vi "Lab Panel V6.00.vi"() -> ()   [LabVIEW 2017] (continued)
                  tunnel: [w1483 w1515] -> w1477
                  tunnel: w1475 -> [_ w1514]
                  tunnel: w1474 -> [_ w1513]
                  tunnel: w1473 -> [_ w1512]
                  tunnel: w1472 -> [_ w1510]
                  frame False {
                    # "stop test"
                    n865 = stacked-sequence {
                      tunnel: w1484 -> [w1493 _]
                      tunnel: [w1485 _] -> w1483
                      frame #0 {
                        n866 = local read "DISP LAB03-2"() -> (w1492:T4)
                        n867 = Unbundle(w1492) -> ("CYCLE"=w1490:dbl, "MINS"=w1491:dbl)  [unwired: 1 out]
                        n868 = case shown="\"CYCLE TEST\"" w1493 {
                          tunnel: w1491 -> [_ _ w1500]
                          tunnel: w1490 -> [w1498 w1499 _]
                          tunnel: [w1498 w1499 w1500] -> w1489
                          frame "CHART TEST", Default {
                          }
                          frame "CYCLE TEST" {
                          }
                          frame "T-RISE TEST" {
                          }
                        }
                        n869 = local read "TDMS LAB03-2"() -> (w1497:refnum<k34>)
                        n870 = Build Array("STOPPED") -> (w1494:string[])
                        n871 = Build Array(w1489) -> (w1488:dbl[])
                        n872 = TDMS Write(0:w1497, 5:"TEST RESULT", 7:w1494, 9:w1488) -> (4:w1486:refnum<k34>, 15:w1487:errorcluster)  [unwired: 2 in, 2 out]
                        n873 = TDMS Close(8:w1487, 11:w1486) -> (0:w1485:errorcluster)  [unwired: 1 out]
                      }
                      frame #1 {
                        n874 = local read "DISP LAB03-2"() -> (w1504:T4)
                        n875 = stacked-sequence {
                          tunnel: "LAB03-2" -> [w1506 w1508]
                          frame #0 {
                            n876 = call "sub vi - defrag tdms v1.vi"("panel id"=w1506) -> ("error out"=w1505:errorcluster)  [unwired: 10 in]
                            n877 = local write "data file error"(w1505) -> ()
                          }
                          frame #1 {
                            n878 = call "Save data file (stop) v3.vi"("panel id"=w1508) -> ("network file save error"=w1507:errorcluster)  [unwired: 9 in, 1 out]
                            n879 = local write "RESULT LAB03-2"(FALSE) -> ()
                            n880 = local write "data file error"(w1507) -> ()
                          }
                        }
                        n881 = Bundle(cluster=w1504, "STATUS"="STOP") -> (w1502:T4)  [unwired: 2 in]
                        n882 = local write "DISP LAB03-2"(w1502) -> ()
                      }
                    }
                  }
                  frame True {
                    n883 = local read "SIG LAB03-2"() -> (w1511:T2)
                    n884 = stacked-sequence {
                      seq-local: [w1522 _] -> [_ w1526]
                      tunnel: w1520 -> [_ w1536]
                      tunnel: w1519 -> [_ w1535]
                      tunnel: w1518 -> [_ w1534]
                      tunnel: w1517 -> [_ w1533]
                      tunnel: w1516 -> [_ w1532]
                      tunnel: [_ w1531] -> w1515
                      tunnel: w1514 -> [_ w1530]
                      tunnel: w1513 -> [_ w1529]
                      tunnel: w1512 -> [_ w1528]
                      tunnel: w1511 -> [w1521 w1527]
                      tunnel: w1510 -> [_ w1525]
                      frame #0 {
                        n885 = Unbundle(w1521) -> ("AMPS"=w1524:dbl)  [unwired: 4 out]
                        n886 = call "Check For Amps on v1.vi"("ID"="LAB03-2", "amps"=w1524) -> ("amps"=w1522:bool)  [unwired: 9 in]
                      }
                      frame #1 {
                        n887 = case shown="True" w1526 {
                          tunnel: w1536 -> [_ w1549]
                          tunnel: w1535 -> [_ w1548]
                          tunnel: w1534 -> [_ w1547]
                          tunnel: w1533 -> [_ w1546]
                          tunnel: w1532 -> [_ w1545]
                          tunnel: [errorcluster {"status"=FALSE, "code"=0, "source"=""} ("error out") w1544] -> w1531
                          tunnel: w1530 -> [_ w1543]
                          tunnel: w1529 -> [_ w1542]
                          tunnel: w1528 -> [_ w1541]
                          tunnel: w1527 -> [_ w1540]
                          tunnel: w1525 -> [_ w1539]
                          frame False {
                            w1537 = FALSE
                            n888 = local write "RUN LAB03-2"(w1537) -> ()
                            n889 = local write "run lab03-2"(w1537) -> ()
                          }
                          frame True {
                            n890 = stacked-sequence {
                              seq-local: [w1550 _ _ _ _] -> [_ w1574 _ _ _]
                              tunnel: w1549 -> [w1555 _ _ _ _]
                              tunnel: w1548 -> [w1552 _ _ _ _]
                              tunnel: w1547 -> [w1565 _ _ _ _]
                              tunnel: w1546 -> [w1558 _ _ _ _]
                              tunnel: w1545 -> [w1553 _ _ _ _]
                              tunnel: [_ w1569 _ _ _] -> w1544
                              tunnel: w1543 -> [_ _ _ w1595 _]
                              tunnel: w1542 -> [_ _ _ w1594 _]
                              tunnel: w1541 -> [_ _ _ w1593 _]
                              tunnel: w1540 -> [_ _ _ _ _]
                              tunnel: w1539 -> [_ _ _ _ w1609]
                              frame #0 {
                                w1551 = "\\"
                                n891 = local read "SET LAB03-2"() -> (w1560:T5)
                                n892 = case shown="\"T-RISE TEST\"" w1565 {
                                tunnel: ["L03-2-CHART TEST-" "L03-2-CYCLE TEST-" "L03-2-T-RISE TEST-"] -> w1561
                                frame "CHART TEST", Default {
                                }
                                frame "CYCLE TEST" {
                                }
                                frame "T-RISE TEST" {
                                }
                                }
                                n893 = Unbundle(w1560) -> ("DESCRIPTION"=w1559:string)  [unwired: 4 out]
                                n894 = Concatenate Strings(w1555, "\\", w1553, w1551, w1552, w1551) -> (w1562:string)
                                n895 = String To Path(string=w1562) -> (path=w1564:path)
                                n896 = Concatenate Strings(w1562, w1561, w1559, "-", w1558, ".tdms") -> (w1550:string)
                                n897 = Create Folder(path (use dialog)=w1564) -> (error out=w1563:errorcluster)  [unwired: 2 in, 2 out]
                                n898 = global write "Global 1.vi" "LAB03-2 FILE"(w1550) -> ()
                                n899 = call <vilib>:"Clear Errors.vi"("error in (no error)"=w1563) -> ()  [unwired: 5 in, 2 out]
                              }
                              frame #1 {
                                (unwired) FALSE
                                n900 = String To Path(string=w1574) -> (path=w1570:path)
                                n901 = TDMS Open(6:FALSE, 10:T22."create or replace" ("operation (0:open)"), 11:w1570) -> (0:w1569:errorcluster, 3:→"TDMS LAB03-2":refnum<k34>)  [unwired: 4 in]
                              }
                              frame #2 {
                                n902 = local read "SET LAB03-2"() -> (w1580:T5)
                                n903 = local read "TDMS LAB03-2"() -> (w1591:refnum<k34>)
                                n904 = Build Array("Testers Name", "Description", "Set Test Cycles", "T-Rise minutes", "T-Rise Deg C") -> (w1581:string[])
                                n905 = Unbundle(w1580) -> ("NAME"=w1579:string, "DESCRIPTION"=w1578:string, "CYCLES"=w1577:dbl, "T-RISE mins"=w1576:dbl, "T-RISE deg C"=w1575:dbl)
                                n906 = Number To Decimal String(number=w1577) -> (decimal integer string=w1590:string)  [unwired: 1 in]
                                n907 = Number To Decimal String(number=w1576) -> (decimal integer string=w1589:string)  [unwired: 1 in]
                                n908 = Number To Decimal String(number=w1575) -> (decimal integer string=w1588:string)  [unwired: 1 in]
                                n909 = Build Array(w1579, w1578, w1590, w1589, w1588) -> (w1587:string[])
                                n910 = TDMS Set Properties(5:w1587, 7:w1581, 11:w1591) -> ()  [unwired: 3 in, 4 out]
                              }
                              frame #3 {
                                n911 = local read "DISP LAB03-2"() -> (w1596:T4)
                                n912 = Concatenate Strings("LAB03-2  ", w1595) -> (w1597:string)
                                n913 = Two Button Dialog(message=w1597, 1:w1593, 2:w1594) -> (T button?=w1599:bool)
                                n914 = case shown="True" w1599 {
                                tunnel: w1596 -> [w1606 w1607]
                                tunnel: [w1606 w1607] -> w1603
                                tunnel: [w1605 w1608] -> w1602
                                tunnel: [w1604 w1608] -> w1601
                                frame False {
                                n915 = Unbundle(w1606) -> ("CYCLE"=w1605:dbl, "MINS"=w1604:dbl)  [unwired: 1 out]
                                }
                                frame True {
                                w1608 = 0.0
                                }
                                }
                                n916 = Bundle(cluster=w1603, "CYCLE"=w1602, "MINS"=w1601, "STATUS"="RUN") -> (w1592:T4)
                                n917 = local write "DISP LAB03-2"(w1592) -> ()
                              }
                              frame #4 {
                                n918 = local read "TEMP START LAB03-2"() -> (w1611:cluster{"TL":dbl, "TN":dbl})
                                n919 = Bundle(cluster=w1611, "TL"=w1609, "TN"=w1609) -> (w1610:cluster{"TL":dbl, "TN":dbl})
                                n920 = local write "TEMP START LAB03-2"(w1610) -> ()
                              }
                            }
                          }
                        }
                      }
                    }
                  }
                }
              }
              event "RUN LAB04-1": Value Change {
                n921 = event-data() -> ("NewVal"=w1616:bool)  [unwired: 1 in, 5 out]
                n922 = local write "run lab04-1"(w1616) -> ()
                n923 = case shown="True" w1616 {
                  tunnel: w1622 -> [_ w1660]
                  tunnel: w1621 -> [_ w1659]
                  tunnel: w1619 -> [w1624 w1658]
                  tunnel: w1620 -> [_ w1657]
                  tunnel: w1618 -> [_ w1656]
                  tunnel: [w1623 w1655] -> w1617
                  tunnel: w1615 -> [_ w1654]
                  tunnel: w1614 -> [_ w1653]
                  tunnel: w1613 -> [_ w1652]
                  tunnel: w1612 -> [_ w1650]
                  frame False {
                    # "stop test"
                    n924 = stacked-sequence {
                      tunnel: w1624 -> [w1633 _]
                      tunnel: [w1625 _] -> w1623
                      frame #0 {
                        n925 = local read "DISP LAB04-1"() -> (w1632:T4)
                        n926 = Unbundle(w1632) -> ("CYCLE"=w1630:dbl, "MINS"=w1631:dbl)  [unwired: 1 out]
                        n927 = case shown="\"CYCLE TEST\"" w1633 {
                          tunnel: w1631 -> [_ _ w1640]
                          tunnel: w1630 -> [w1638 w1639 _]
                          tunnel: [w1638 w1639 w1640] -> w1629
                          frame "CHART TEST", Default {
                          }
                          frame "CYCLE TEST" {
                          }
                          frame "T-RISE TEST" {
                          }
                        }
                        n928 = local read "TDMS LAB04-1"() -> (w1637:refnum<k34>)
                        n929 = Build Array("STOPPED") -> (w1634:string[])
                        n930 = Build Array(w1629) -> (w1628:dbl[])
                        n931 = TDMS Write(0:w1637, 5:"TEST RESULT", 7:w1634, 9:w1628) -> (4:w1626:refnum<k34>, 15:w1627:errorcluster)  [unwired: 2 in, 2 out]
                        n932 = TDMS Close(8:w1627, 11:w1626) -> (0:w1625:errorcluster)  [unwired: 1 out]
                      }
                      frame #1 {
                        n933 = local read "DISP LAB04-1"() -> (w1644:T4)
                        n934 = stacked-sequence {
                          tunnel: "LAB04-1" -> [w1646 w1648]
                          frame #0 {
                            n935 = call "sub vi - defrag tdms v1.vi"("panel id"=w1646) -> ("error out"=w1645:errorcluster)  [unwired: 10 in]
                            n936 = local write "data file error"(w1645) -> ()
                          }
                          frame #1 {
                            n937 = call "Save data file (stop) v3.vi"("panel id"=w1648) -> ("network file save error"=w1647:errorcluster)  [unwired: 9 in, 1 out]
                            n938 = local write "RESULT LAB04-1"(FALSE) -> ()
                            n939 = local write "data file error"(w1647) -> ()
                          }
                        }
                        n940 = Bundle(cluster=w1644, "STATUS"="STOP") -> (w1642:T4)  [unwired: 2 in]
                        n941 = local write "DISP LAB04-1"(w1642) -> ()
                      }
                    }
                  }
                  frame True {
                    n942 = local read "SIG LAB04-1"() -> (w1651:T2)
                    n943 = stacked-sequence {
                      seq-local: [w1662 _] -> [_ w1666]
                      tunnel: w1660 -> [_ w1676]
                      tunnel: w1659 -> [_ w1675]
                      tunnel: w1658 -> [_ w1674]
                      tunnel: w1657 -> [_ w1673]
                      tunnel: w1656 -> [_ w1672]
                      tunnel: [_ w1671] -> w1655
                      tunnel: w1654 -> [_ w1670]
                      tunnel: w1653 -> [_ w1669]
                      tunnel: w1652 -> [_ w1668]
                      tunnel: w1651 -> [w1661 w1667]
                      tunnel: w1650 -> [_ w1665]
                      frame #0 {
                        n944 = Unbundle(w1661) -> ("AMPS"=w1664:dbl)  [unwired: 4 out]
                        n945 = call "Check For Amps on v1.vi"("ID"="LAB04-1", "amps"=w1664) -> ("amps"=w1662:bool)  [unwired: 9 in]
                      }
                      frame #1 {
                        n946 = case shown="True" w1666 {
                          tunnel: w1676 -> [_ w1689]
                          tunnel: w1675 -> [_ w1688]
                          tunnel: w1674 -> [_ w1687]
                          tunnel: w1673 -> [_ w1686]
                          tunnel: w1672 -> [_ w1685]
                          tunnel: [errorcluster {"status"=FALSE, "code"=0, "source"=""} ("error out") w1684] -> w1671
                          tunnel: w1670 -> [_ w1683]
                          tunnel: w1669 -> [_ w1682]
                          tunnel: w1668 -> [_ w1681]
                          tunnel: w1667 -> [_ w1680]
                          tunnel: w1665 -> [_ w1679]
                          frame False {
                            w1677 = FALSE
                            n947 = local write "RUN LAB04-1"(w1677) -> ()
                            n948 = local write "run lab04-1"(w1677) -> ()
                          }
                          frame True {
                            n949 = stacked-sequence {
                              seq-local: [w1690 _ _ _ _] -> [_ w1714 _ _ _]
                              tunnel: w1689 -> [w1695 _ _ _ _]
                              tunnel: w1688 -> [w1691 _ _ _ _]
                              tunnel: w1687 -> [w1705 _ _ _ _]
                              tunnel: w1686 -> [w1698 _ _ _ _]
                              tunnel: w1685 -> [w1693 _ _ _ _]
                              tunnel: [_ w1709 _ _ _] -> w1684
                              tunnel: w1683 -> [_ _ _ w1735 _]
                              tunnel: w1682 -> [_ _ _ w1734 _]
                              tunnel: w1681 -> [_ _ _ w1733 _]
                              tunnel: w1680 -> [_ _ _ _ _]
                              tunnel: w1679 -> [_ _ _ _ w1749]
                              frame #0 {
                                w1692 = "\\"
                                n950 = local read "SET LAB04-1"() -> (w1700:T5)
                                n951 = case shown="\"CYCLE TEST\"" w1705 {
                                tunnel: ["L04-1-CHART TEST-" "L04-1-CYCLE TEST-" "L04-1-T-RISE TEST-"] -> w1701
                                frame "CHART TEST", Default {
                                }
                                frame "CYCLE TEST" {
                                }
                                frame "T-RISE TEST" {
                                }
                                }
                                n952 = Unbundle(w1700) -> ("DESCRIPTION"=w1699:string)  [unwired: 4 out]
                                n953 = Concatenate Strings(w1695, "\\", w1693, w1692, w1691, w1692) -> (w1702:string)
                                n954 = String To Path(string=w1702) -> (path=w1704:path)
                                n955 = Concatenate Strings(w1702, w1701, w1699, "-", w1698, ".tdms") -> (w1690:string)
                                n956 = Create Folder(path (use dialog)=w1704) -> (error out=w1703:errorcluster)  [unwired: 2 in, 2 out]
                                n957 = global write "Global 1.vi" "LAB04-1 FILE"(w1690) -> ()
                                n958 = call <vilib>:"Clear Errors.vi"("error in (no error)"=w1703) -> ()  [unwired: 5 in, 2 out]
                              }
                              frame #1 {
                                (unwired) FALSE
                                n959 = String To Path(string=w1714) -> (path=w1710:path)
                                n960 = TDMS Open(6:FALSE, 10:T22."create or replace" ("operation (0:open)"), 11:w1710) -> (0:w1709:errorcluster, 3:→"TDMS LAB04-1":refnum<k34>)  [unwired: 4 in]
                              }
                              frame #2 {
                                n961 = local read "SET LAB04-1"() -> (w1720:T5)
                                n962 = local read "TDMS LAB04-1"() -> (w1731:refnum<k34>)
                                n963 = Build Array("Testers Name", "Description", "Set Test Cycles", "T-Rise minutes", "T-Rise Deg C") -> (w1721:string[])
                                n964 = Unbundle(w1720) -> ("NAME"=w1719:string, "DESCRIPTION"=w1718:string, "CYCLES"=w1717:dbl, "T-RISE mins"=w1716:dbl, "T-RISE deg C"=w1715:dbl)
                                n965 = Number To Decimal String(number=w1717) -> (decimal integer string=w1730:string)  [unwired: 1 in]
                                n966 = Number To Decimal String(number=w1716) -> (decimal integer string=w1729:string)  [unwired: 1 in]
                                n967 = Number To Decimal String(number=w1715) -> (decimal integer string=w1728:string)  [unwired: 1 in]
                                n968 = Build Array(w1719, w1718, w1730, w1729, w1728) -> (w1727:string[])
                                n969 = TDMS Set Properties(5:w1727, 7:w1721, 11:w1731) -> ()  [unwired: 3 in, 4 out]
                              }
                              frame #3 {
                                n970 = local read "DISP LAB04-1"() -> (w1736:T4)
                                n971 = Concatenate Strings("LAB04-1  ", w1735) -> (w1737:string)
                                n972 = Two Button Dialog(message=w1737, 1:w1733, 2:w1734) -> (T button?=w1739:bool)
                                n973 = case shown="True" w1739 {
                                tunnel: w1736 -> [w1746 w1747]
                                tunnel: [w1746 w1747] -> w1743
                                tunnel: [w1745 w1748] -> w1742
                                tunnel: [w1744 w1748] -> w1741
                                frame False {
                                n974 = Unbundle(w1746) -> ("CYCLE"=w1745:dbl, "MINS"=w1744:dbl)  [unwired: 1 out]
                                }
                                frame True {
                                w1748 = 0.0
                                }
                                }
                                n975 = Bundle(cluster=w1743, "CYCLE"=w1742, "MINS"=w1741, "STATUS"="RUN") -> (w1732:T4)
                                n976 = local write "DISP LAB04-1"(w1732) -> ()
                              }
                              frame #4 {
                                n977 = local read "TEMP START LAB04-1"() -> (w1751:cluster{"TL":dbl, "TN":dbl})
                                n978 = Bundle(cluster=w1751, "TL"=w1749, "TN"=w1749) -> (w1750:cluster{"TL":dbl, "TN":dbl})
                                n979 = local write "TEMP START LAB04-1"(w1750) -> ()
                              }
                            }
                          }
                        }
                      }
                    }
                  }
                }
              }
              event "RUN LAB04-2": Value Change {
                n980 = event-data() -> ("NewVal"=w1756:bool)  [unwired: 1 in, 5 out]
                n981 = local write "run lab04-2"(w1756) -> ()
                n982 = case shown="True" w1756 {
                  tunnel: w1762 -> [_ w1800]
                  tunnel: w1761 -> [_ w1799]
                  tunnel: w1759 -> [w1764 w1798]
                  tunnel: w1760 -> [_ w1797]
                  tunnel: w1758 -> [_ w1796]
                  tunnel: [w1763 w1795] -> w1757
                  tunnel: w1755 -> [_ w1794]
                  tunnel: w1754 -> [_ w1793]
                  tunnel: w1753 -> [_ w1792]
                  tunnel: w1752 -> [_ w1790]
                  frame False {
                    # "stop test"
                    n983 = stacked-sequence {
                      tunnel: w1764 -> [w1773 _]
                      tunnel: [w1765 _] -> w1763
                      frame #0 {
                        n984 = local read "DISP LAB04-2"() -> (w1772:T4)
                        n985 = Unbundle(w1772) -> ("CYCLE"=w1770:dbl, "MINS"=w1771:dbl)  [unwired: 1 out]
                        n986 = case shown="\"CYCLE TEST\"" w1773 {
                          tunnel: w1771 -> [_ _ w1780]
                          tunnel: w1770 -> [w1778 w1779 _]
                          tunnel: [w1778 w1779 w1780] -> w1769
                          frame "CHART TEST", Default {
                          }
                          frame "CYCLE TEST" {
                          }
                          frame "T-RISE TEST" {
                          }
                        }
                        n987 = local read "TDMS LAB04-2"() -> (w1777:refnum<k34>)
                        n988 = Build Array("STOPPED") -> (w1774:string[])
                        n989 = Build Array(w1769) -> (w1768:dbl[])
                        n990 = TDMS Write(0:w1777, 5:"TEST RESULT", 7:w1774, 9:w1768) -> (4:w1766:refnum<k34>, 15:w1767:errorcluster)  [unwired: 2 in, 2 out]
                        n991 = TDMS Close(8:w1767, 11:w1766) -> (0:w1765:errorcluster)  [unwired: 1 out]
                      }
                      frame #1 {
                        n992 = local read "DISP LAB04-2"() -> (w1784:T4)
                        n993 = stacked-sequence {
                          tunnel: "LAB04-2" -> [w1786 w1788]
                          frame #0 {
                            n994 = call "sub vi - defrag tdms v1.vi"("panel id"=w1786) -> ("error out"=w1785:errorcluster)  [unwired: 10 in]
                            n995 = local write "data file error"(w1785) -> ()
                          }
                          frame #1 {
                            n996 = call "Save data file (stop) v3.vi"("panel id"=w1788) -> ("network file save error"=w1787:errorcluster)  [unwired: 9 in, 1 out]
                            n997 = local write "RESULT LAB04-2"(FALSE) -> ()
                            n998 = local write "data file error"(w1787) -> ()
                          }
                        }
                        n999 = Bundle(cluster=w1784, "STATUS"="STOP") -> (w1782:T4)  [unwired: 2 in]
                        n1000 = local write "DISP LAB04-2"(w1782) -> ()
                      }
                    }
                  }
                  frame True {
                    n1001 = local read "SIG LAB04-2"() -> (w1791:T2)
                    n1002 = stacked-sequence {
                      seq-local: [w1802 _] -> [_ w1806]
                      tunnel: w1800 -> [_ w1816]
                      tunnel: w1799 -> [_ w1815]
                      tunnel: w1798 -> [_ w1814]
                      tunnel: w1797 -> [_ w1813]
                      tunnel: w1796 -> [_ w1812]
                      tunnel: [_ w1811] -> w1795
                      tunnel: w1794 -> [_ w1810]
                      tunnel: w1793 -> [_ w1809]
                      tunnel: w1792 -> [_ w1808]
                      tunnel: w1791 -> [w1801 w1807]
                      tunnel: w1790 -> [_ w1805]
                      frame #0 {
                        n1003 = Unbundle(w1801) -> ("AMPS"=w1804:dbl)  [unwired: 4 out]
                        n1004 = call "Check For Amps on v1.vi"("ID"="LAB04-2", "amps"=w1804) -> ("amps"=w1802:bool)  [unwired: 9 in]
                      }
                      frame #1 {
                        n1005 = case shown="True" w1806 {
                          tunnel: w1816 -> [_ w1829]
                          tunnel: w1815 -> [_ w1828]
                          tunnel: w1814 -> [_ w1827]
                          tunnel: w1813 -> [_ w1826]
                          tunnel: w1812 -> [_ w1825]
                          tunnel: [errorcluster {"status"=FALSE, "code"=0, "source"=""} ("error out") w1824] -> w1811
                          tunnel: w1810 -> [_ w1823]
                          tunnel: w1809 -> [_ w1822]
                          tunnel: w1808 -> [_ w1821]
                          tunnel: w1807 -> [_ w1820]
                          tunnel: w1805 -> [_ w1819]
                          frame False {
                            w1817 = FALSE
                            n1006 = local write "RUN LAB04-2"(w1817) -> ()
                            n1007 = local write "run lab04-2"(w1817) -> ()
                          }
                          frame True {
                            n1008 = stacked-sequence {
                              seq-local: [w1830 _ _ _ _] -> [_ w1854 _ _ _]
                              tunnel: w1829 -> [w1835 _ _ _ _]
                              tunnel: w1828 -> [w1831 _ _ _ _]
                              tunnel: w1827 -> [w1845 _ _ _ _]
                              tunnel: w1826 -> [w1838 _ _ _ _]
                              tunnel: w1825 -> [w1833 _ _ _ _]
                              tunnel: [_ w1849 _ _ _] -> w1824
                              tunnel: w1823 -> [_ _ _ w1875 _]
                              tunnel: w1822 -> [_ _ _ w1874 _]
                              tunnel: w1821 -> [_ _ _ w1873 _]
                              tunnel: w1820 -> [_ _ _ _ _]
                              tunnel: w1819 -> [_ _ _ _ w1889]
                              frame #0 {
                                w1832 = "\\"
                                n1009 = local read "SET LAB04-2"() -> (w1840:T5)
                                n1010 = case shown="\"CHART TEST\", Default" w1845 {
                                tunnel: ["L04-2-CHART TEST-" "L04-2-CYCLE TEST-" "L04-2-T-RISE TEST-"] -> w1841
                                frame "CHART TEST", Default {
                                }
                                frame "CYCLE TEST" {
                                }
                                frame "T-RISE TEST" {
                                }
                                }
                                n1011 = Unbundle(w1840) -> ("DESCRIPTION"=w1839:string)  [unwired: 4 out]
                                n1012 = Concatenate Strings(w1835, "\\", w1833, w1832, w1831, w1832) -> (w1842:string)
                                n1013 = String To Path(string=w1842) -> (path=w1844:path)
                                n1014 = Concatenate Strings(w1842, w1841, w1839, "-", w1838, ".tdms") -> (w1830:string)
                                n1015 = Create Folder(path (use dialog)=w1844) -> (error out=w1843:errorcluster)  [unwired: 2 in, 2 out]
                                n1016 = global write "Global 1.vi" "LAB04-2 FILE"(w1830) -> ()
                                n1017 = call <vilib>:"Clear Errors.vi"("error in (no error)"=w1843) -> ()  [unwired: 5 in, 2 out]
                              }
                              frame #1 {
                                (unwired) FALSE
                                n1018 = String To Path(string=w1854) -> (path=w1850:path)
                                n1019 = TDMS Open(6:FALSE, 10:T22."create or replace" ("operation (0:open)"), 11:w1850) -> (0:w1849:errorcluster, 3:→"TDMS LAB04-2":refnum<k34>)  [unwired: 4 in]
                              }
                              frame #2 {
                                n1020 = local read "SET LAB04-2"() -> (w1860:T5)
                                n1021 = local read "TDMS LAB04-2"() -> (w1871:refnum<k34>)
                                n1022 = Build Array("Testers Name", "Description", "Set Test Cycles", "T-Rise minutes", "T-Rise Deg C") -> (w1861:string[])
                                n1023 = Unbundle(w1860) -> ("NAME"=w1859:string, "DESCRIPTION"=w1858:string, "CYCLES"=w1857:dbl, "T-RISE mins"=w1856:dbl, "T-RISE deg C"=w1855:dbl)
                                n1024 = Number To Decimal String(number=w1857) -> (decimal integer string=w1870:string)  [unwired: 1 in]
                                n1025 = Number To Decimal String(number=w1856) -> (decimal integer string=w1869:string)  [unwired: 1 in]
                                n1026 = Number To Decimal String(number=w1855) -> (decimal integer string=w1868:string)  [unwired: 1 in]
                                n1027 = Build Array(w1859, w1858, w1870, w1869, w1868) -> (w1867:string[])
                                n1028 = TDMS Set Properties(5:w1867, 7:w1861, 11:w1871) -> ()  [unwired: 3 in, 4 out]
                              }
                              frame #3 {
                                n1029 = local read "DISP LAB04-2"() -> (w1876:T4)
                                n1030 = Concatenate Strings("LAB04-2 ", w1875) -> (w1877:string)
                                n1031 = Two Button Dialog(message=w1877, 1:w1873, 2:w1874) -> (T button?=w1879:bool)
                                n1032 = case shown="True" w1879 {
                                tunnel: w1876 -> [w1886 w1887]
                                tunnel: [w1886 w1887] -> w1883
                                tunnel: [w1885 w1888] -> w1882
                                tunnel: [w1884 w1888] -> w1881
                                frame False {
                                n1033 = Unbundle(w1886) -> ("CYCLE"=w1885:dbl, "MINS"=w1884:dbl)  [unwired: 1 out]
                                }
                                frame True {
                                w1888 = 0.0
                                }
                                }
                                n1034 = Bundle(cluster=w1883, "CYCLE"=w1882, "MINS"=w1881, "STATUS"="RUN") -> (w1872:T4)
                                n1035 = local write "DISP LAB04-2"(w1872) -> ()
                              }
                              frame #4 {
                                n1036 = local read "TEMP START LAB04-2"() -> (w1891:cluster{"TL":dbl, "TN":dbl})
                                n1037 = Bundle(cluster=w1891, "TL"=w1889, "TN"=w1889) -> (w1890:cluster{"TL":dbl, "TN":dbl})
                                n1038 = local write "TEMP START LAB04-2"(w1890) -> ()
                              }
                            }
                          }
                        }
                      }
                    }
                  }
                }
              }
              event "RUN LAB05-1": Value Change {
                n1039 = event-data() -> ("NewVal"=w1896:bool)  [unwired: 1 in, 5 out]
                n1040 = local write "run lab05-1"(w1896) -> ()
                n1041 = case shown="True" w1896 {
                  tunnel: w1902 -> [_ w1940]
                  tunnel: w1901 -> [_ w1939]
                  tunnel: w1899 -> [w1904 w1938]
                  tunnel: w1900 -> [_ w1937]
                  tunnel: w1898 -> [_ w1936]
                  tunnel: [w1903 w1935] -> w1897
                  tunnel: w1895 -> [_ w1934]
                  tunnel: w1894 -> [_ w1933]
                  tunnel: w1893 -> [_ w1932]
                  tunnel: w1892 -> [_ w1930]
                  frame False {
                    # "stop test"
                    n1042 = stacked-sequence {
                      tunnel: w1904 -> [w1913 _]
                      tunnel: [w1905 _] -> w1903
                      frame #0 {
                        n1043 = local read "DISP LAB05-1"() -> (w1912:T4)
                        n1044 = Unbundle(w1912) -> ("CYCLE"=w1910:dbl, "MINS"=w1911:dbl)  [unwired: 1 out]
                        n1045 = case shown="\"CYCLE TEST\"" w1913 {
                          tunnel: w1911 -> [_ _ w1920]
                          tunnel: w1910 -> [w1918 w1919 _]
                          tunnel: [w1918 w1919 w1920] -> w1909
                          frame "CHART TEST", Default {
                          }
                          frame "CYCLE TEST" {
                          }
                          frame "T-RISE TEST" {
                          }
                        }
                        n1046 = local read "TDMS LAB05-1"() -> (w1917:refnum<k34>)
                        n1047 = Build Array("STOPPED") -> (w1914:string[])
                        n1048 = Build Array(w1909) -> (w1908:dbl[])
                        n1049 = TDMS Write(0:w1917, 5:"TEST RESULT", 7:w1914, 9:w1908) -> (4:w1906:refnum<k34>, 15:w1907:errorcluster)  [unwired: 2 in, 2 out]
                        n1050 = TDMS Close(8:w1907, 11:w1906) -> (0:w1905:errorcluster)  [unwired: 1 out]
                      }
                      frame #1 {
                        n1051 = local read "DISP LAB05-1"() -> (w1924:T4)
                        n1052 = stacked-sequence {
                          tunnel: "LAB05-1" -> [w1926 w1928]
                          frame #0 {
                            n1053 = call "sub vi - defrag tdms v1.vi"("panel id"=w1926) -> ("error out"=w1925:errorcluster)  [unwired: 10 in]
                            n1054 = local write "data file error"(w1925) -> ()
                          }
                          frame #1 {
                            n1055 = call "Save data file (stop) v3.vi"("panel id"=w1928) -> ("network file save error"=w1927:errorcluster)  [unwired: 9 in, 1 out]
                            n1056 = local write "RESULT LAB05-1"(FALSE) -> ()
                            n1057 = local write "data file error"(w1927) -> ()
                          }
                        }
                        n1058 = Bundle(cluster=w1924, "STATUS"="STOP") -> (w1922:T4)  [unwired: 2 in]
                        n1059 = local write "DISP LAB05-1"(w1922) -> ()
                      }
                    }
                  }
                  frame True {
                    n1060 = local read "SIG LAB05-1"() -> (w1931:T2)
                    n1061 = stacked-sequence {
                      seq-local: [w1942 _] -> [_ w1946]
                      tunnel: w1940 -> [_ w1956]
                      tunnel: w1939 -> [_ w1955]
                      tunnel: w1938 -> [_ w1954]
                      tunnel: w1937 -> [_ w1953]
                      tunnel: w1936 -> [_ w1952]
                      tunnel: [_ w1951] -> w1935
                      tunnel: w1934 -> [_ w1950]
                      tunnel: w1933 -> [_ w1949]
                      tunnel: w1932 -> [_ w1948]
                      tunnel: w1931 -> [w1941 w1947]
                      tunnel: w1930 -> [_ w1945]
                      frame #0 {
                        n1062 = Unbundle(w1941) -> ("AMPS"=w1944:dbl)  [unwired: 4 out]
                        n1063 = call "Check For Amps on v1.vi"("ID"="LAB05-1", "amps"=w1944) -> ("amps"=w1942:bool)  [unwired: 9 in]
                      }
                      frame #1 {
                        n1064 = case shown="True" w1946 {
                          tunnel: w1956 -> [_ w1969]
                          tunnel: w1955 -> [_ w1968]
                          tunnel: w1954 -> [_ w1967]
                          tunnel: w1953 -> [_ w1966]
                          tunnel: w1952 -> [_ w1965]
                          tunnel: [errorcluster {"status"=FALSE, "code"=0, "source"=""} ("error out") w1964] -> w1951
                          tunnel: w1950 -> [_ w1963]
                          tunnel: w1949 -> [_ w1962]
                          tunnel: w1948 -> [_ w1961]
                          tunnel: w1947 -> [_ w1960]
                          tunnel: w1945 -> [_ w1959]
                          frame False {
                            w1957 = FALSE
                            n1065 = local write "RUN LAB05-1"(w1957) -> ()
                            n1066 = local write "run lab05-1"(w1957) -> ()
                          }
                          frame True {
                            n1067 = stacked-sequence {
                              seq-local: [w1970 _ _ _ _] -> [_ w1994 _ _ _]
                              tunnel: w1969 -> [w1975 _ _ _ _]
                              tunnel: w1968 -> [w1971 _ _ _ _]
                              tunnel: w1967 -> [w1985 _ _ _ _]
                              tunnel: w1966 -> [w1978 _ _ _ _]
                              tunnel: w1965 -> [w1973 _ _ _ _]
                              tunnel: [_ w1989 _ _ _] -> w1964
                              tunnel: w1963 -> [_ _ _ w2014 _]
                              tunnel: w1962 -> [_ _ _ w2013 _]
                              tunnel: w1961 -> [_ _ _ w2012 _]
                              tunnel: w1960 -> [_ _ _ _ _]
                              tunnel: w1959 -> [_ _ _ _ w2029]
                              frame #0 {
                                w1972 = "\\"
                                n1068 = local read "SET LAB05-1"() -> (w1980:T5)
                                n1069 = case shown="\"CYCLE TEST\"" w1985 {
                                tunnel: ["L05-1-CHART TEST-" "L05-1-CYCLE TEST-" "L05-1-T-RISE TEST-"] -> w1981
                                frame "CHART TEST", Default {
                                }
                                frame "CYCLE TEST" {
                                }
                                frame "T-RISE TEST" {
                                }
                                }
                                n1070 = Unbundle(w1980) -> ("DESCRIPTION"=w1979:string)  [unwired: 4 out]
                                n1071 = Concatenate Strings(w1975, "\\", w1973, w1972, w1971, w1972) -> (w1982:string)
                                n1072 = String To Path(string=w1982) -> (path=w1984:path)
                                n1073 = Concatenate Strings(w1982, w1981, w1979, "-", w1978, ".tdms") -> (w1970:string)
                                n1074 = Create Folder(path (use dialog)=w1984) -> (error out=w1983:errorcluster)  [unwired: 2 in, 2 out]
                                n1075 = global write "Global 1.vi" "LAB05-1 FILE"(w1970) -> ()
                                n1076 = call <vilib>:"Clear Errors.vi"("error in (no error)"=w1983) -> ()  [unwired: 5 in, 2 out]
                              }
                              frame #1 {
                                (unwired) FALSE
                                n1077 = String To Path(string=w1994) -> (path=w1990:path)
                                n1078 = TDMS Open(6:FALSE, 10:T22."create or replace" ("operation (0:open)"), 11:w1990) -> (0:w1989:errorcluster, 3:→"TDMS LAB05-1":refnum<k34>)  [unwired: 4 in]
                              }
                              frame #2 {
                                n1079 = local read "SET LAB05-1"() -> (w2000:T5)
                                n1080 = local read "TDMS LAB05-1"() -> (w2011:refnum<k34>)
                                n1081 = Build Array("Testers Name", "Description", "Set Test Cycles", "T-Rise minutes", "T-Rise Deg C") -> (w2001:string[])
                                n1082 = Unbundle(w2000) -> ("NAME"=w1999:string, "DESCRIPTION"=w1998:string, "CYCLES"=w1997:dbl, "T-RISE mins"=w1996:dbl, "T-RISE deg C"=w1995:dbl)
                                n1083 = Number To Decimal String(number=w1997) -> (decimal integer string=w2010:string)  [unwired: 1 in]
                                n1084 = Number To Decimal String(number=w1996) -> (decimal integer string=w2009:string)  [unwired: 1 in]
                                n1085 = Number To Decimal String(number=w1995) -> (decimal integer string=w2008:string)  [unwired: 1 in]
                                n1086 = Build Array(w1999, w1998, w2010, w2009, w2008) -> (w2007:string[])
                                n1087 = TDMS Set Properties(5:w2007, 7:w2001, 11:w2011) -> ()  [unwired: 3 in, 4 out]
                              }
                              frame #3 {
                                n1088 = local read "DISP LAB05-1"() -> (w2016:T4)
                                n1089 = Concatenate Strings("LAB05-1  ", w2014) -> (w2017:string)
                                n1090 = Two Button Dialog(message=w2017, 1:w2012, 2:w2013) -> (T button?=w2019:bool)
                                n1091 = case shown="True" w2019 {
                                tunnel: w2016 -> [w2026 w2027]
                                tunnel: [w2026 w2027] -> w2023
                                tunnel: [w2025 w2028] -> w2022
                                tunnel: [w2024 w2028] -> w2021
                                frame False {
                                n1092 = Unbundle(w2026) -> ("CYCLE"=w2025:dbl, "MINS"=w2024:dbl)  [unwired: 1 out]
                                }
                                frame True {
                                w2028 = 0.0
                                }
                                }
                                n1093 = Bundle(cluster=w2023, "CYCLE"=w2022, "MINS"=w2021, "STATUS"="RUN") -> (w2015:T4)
                                n1094 = local write "DISP LAB05-1"(w2015) -> ()
                              }
                              frame #4 {
                                n1095 = local read "TEMP START LAB05-1"() -> (w2031:cluster{"TL":dbl, "TN":dbl})
                                n1096 = Bundle(cluster=w2031, "TL"=w2029, "TN"=w2029) -> (w2030:cluster{"TL":dbl, "TN":dbl})
                                n1097 = local write "TEMP START LAB05-1"(w2030) -> ()
                              }
                            }
                          }
                        }
                      }
                    }
                  }
                }
              }
              event "RUN LAB05-2": Value Change {
                n1098 = event-data() -> ("NewVal"=w2037:bool)  [unwired: 1 in, 5 out]
                n1099 = local read "SIG LAB05-2"() -> (w2033:T2)
                n1100 = case shown="True" w2037 {
                  tunnel: w2043 -> [_ w2081]
                  tunnel: w2042 -> [_ w2080]
                  tunnel: w2040 -> [w2045 w2079]
                  tunnel: w2041 -> [_ w2078]
                  tunnel: w2039 -> [_ w2077]
                  tunnel: [w2044 w2076] -> w2038
                  tunnel: w2036 -> [_ w2075]
                  tunnel: w2035 -> [_ w2074]
                  tunnel: w2034 -> [_ w2073]
                  tunnel: w2033 -> [_ w2072]
                  tunnel: w2032 -> [_ w2071]
                  frame False {
                    # "stop test"
                    n1101 = stacked-sequence {
                      tunnel: w2045 -> [w2054 _]
                      tunnel: [w2046 _] -> w2044
                      frame #0 {
                        n1102 = local read "DISP LAB05-2"() -> (w2053:T4)
                        n1103 = Unbundle(w2053) -> ("CYCLE"=w2051:dbl, "MINS"=w2052:dbl)  [unwired: 1 out]
                        n1104 = case shown="\"CYCLE TEST\"" w2054 {
                          tunnel: w2052 -> [_ _ w2061]
                          tunnel: w2051 -> [w2059 w2060 _]
                          tunnel: [w2059 w2060 w2061] -> w2050
                          frame "CHART TEST", Default {
                          }
                          frame "CYCLE TEST" {
                          }
                          frame "T-RISE TEST" {
                          }
                        }
                        n1105 = local read "TDMS LAB05-2"() -> (w2058:refnum<k34>)
                        n1106 = Build Array("STOPPED") -> (w2055:string[])
                        n1107 = Build Array(w2050) -> (w2049:dbl[])
                        n1108 = TDMS Write(0:w2058, 5:"TEST RESULT", 7:w2055, 9:w2049) -> (4:w2047:refnum<k34>, 15:w2048:errorcluster)  [unwired: 2 in, 2 out]
                        n1109 = TDMS Close(8:w2048, 11:w2047) -> (0:w2046:errorcluster)  [unwired: 1 out]
                      }
                      frame #1 {
                        n1110 = local read "DISP LAB05-2"() -> (w2065:T4)
                        n1111 = stacked-sequence {
                          tunnel: "LAB05-2" -> [w2067 w2069]
                          frame #0 {
                            n1112 = call "sub vi - defrag tdms v1.vi"("panel id"=w2067) -> ("error out"=w2066:errorcluster)  [unwired: 10 in]
                            n1113 = local write "data file error"(w2066) -> ()
                          }
                          frame #1 {
                            n1114 = local write "RESULT LAB05-2"(FALSE) -> ()
                            n1115 = call "Save data file (stop) v3.vi"("panel id"=w2069) -> ("network file save error"=w2068:errorcluster)  [unwired: 9 in, 1 out]
                            n1116 = local write "data file error"(w2068) -> ()
                          }
                        }
                        n1117 = Bundle(cluster=w2065, "STATUS"="STOP") -> (w2063:T4)  [unwired: 2 in]
                        n1118 = local write "DISP LAB05-2"(w2063) -> ()
                      }
                    }
                  }
                  frame True {
                    n1119 = stacked-sequence {
                      seq-local: [w2083 _] -> [_ w2087]
                      tunnel: w2081 -> [_ w2097]
                      tunnel: w2080 -> [_ w2096]
                      tunnel: w2079 -> [_ w2095]
                      tunnel: w2078 -> [_ w2094]
                      tunnel: w2077 -> [_ w2093]
                      tunnel: [_ w2092] -> w2076
                      tunnel: w2075 -> [_ w2091]
                      tunnel: w2074 -> [_ w2090]
                      tunnel: w2073 -> [_ w2089]
                      tunnel: w2072 -> [w2082 w2088]
                      tunnel: w2071 -> [_ w2086]
                      frame #0 {
                        n1120 = Unbundle(w2082) -> ("AMPS"=w2085:dbl)  [unwired: 4 out]
                        n1121 = call "Check For Amps on v1.vi"("ID"="LAB05-2", "amps"=w2085) -> ("amps"=w2083:bool)  [unwired: 9 in]
                      }
                      frame #1 {
                        n1122 = case shown="True" w2087 {
                          tunnel: w2097 -> [_ w2109]
                          tunnel: w2096 -> [_ w2107]
                          tunnel: w2095 -> [_ w2104]
                          tunnel: w2094 -> [_ w2105]
                          tunnel: w2093 -> [_ w2108]
                          tunnel: [errorcluster {"status"=FALSE, "code"=0, "source"=""} ("error out") w2100] -> w2092
                          tunnel: w2091 -> [_ w2103]
                          tunnel: w2090 -> [_ w2102]
                          tunnel: w2089 -> [_ w2101]
                          tunnel: w2088 -> [_ w2106]
                          tunnel: w2086 -> [_ w2110]
                          frame False {
                            w2098 = FALSE
                            n1123 = local write "RUN LAB05-2"(w2098) -> ()
                            n1124 = local write "run lab05-2"(w2098) -> ()
                          }
                          frame True {
                            n1125 = stacked-sequence {
                              seq-local: [w2111 _ _ _ _] -> [_ w2135 _ _ _]
                              tunnel: w2109 -> [w2116 _ _ _ _]
                              tunnel: w2107 -> [w2112 _ _ _ _]
                              tunnel: w2104 -> [w2126 _ _ _ _]
                              tunnel: w2105 -> [w2119 _ _ _ _]
                              tunnel: w2108 -> [w2114 _ _ _ _]
                              tunnel: [_ w2130 _ _ _] -> w2100
                              tunnel: w2103 -> [_ _ _ w2155 _]
                              tunnel: w2102 -> [_ _ _ w2154 _]
                              tunnel: w2101 -> [_ _ _ w2153 _]
                              tunnel: w2106 -> [_ _ _ _ _]
                              tunnel: w2110 -> [_ _ _ _ w2170]
                              frame #0 {
                                w2113 = "\\"
                                n1126 = local read "SET LAB05-2"() -> (w2121:T5)
                                n1127 = case shown="\"CYCLE TEST\"" w2126 {
                                tunnel: ["L05-2-CHART TEST-" "L05-2-CYCLE TEST-" "L05-2-T-RISE TEST-"] -> w2122
                                frame "CHART TEST", Default {
                                }
                                frame "CYCLE TEST" {
                                }
                                frame "T-RISE TEST" {
                                }
